vi "Update Command.vi"(6 "Time":dbl, 8 "error in (no error)":errorcluster, 11 "2WayValve in":refnum<class "2WayValveV.lvclass">) -> (0 "error out":errorcluster, 3 "2WayValve out":refnum<class "2WayValveV.lvclass">)   [LabVIEW 2020, in "VolatusGUIElements.lvlib" / "2WayValveV.lvclass"]
uses:
  2WayValveV.lvclass
  2WayValveV.lvclass/2WayValveV.ctl
  lv-vecto/Vecto/Channel DBL/Channel DBL.lvclass/Channel DBL.ctl
  lv-vecto/Vecto/Group DBL/Value by Index.vi
  lv-vecto/Vecto/Channel DBL/Channel DBL.lvclass
  lv-vecto/Vecto/Vecto.lvlib
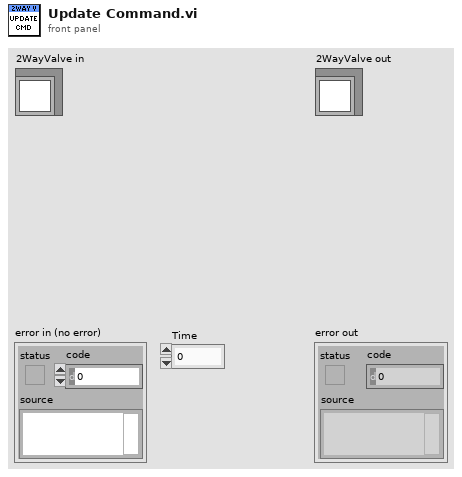
[diagram p1: front panel]
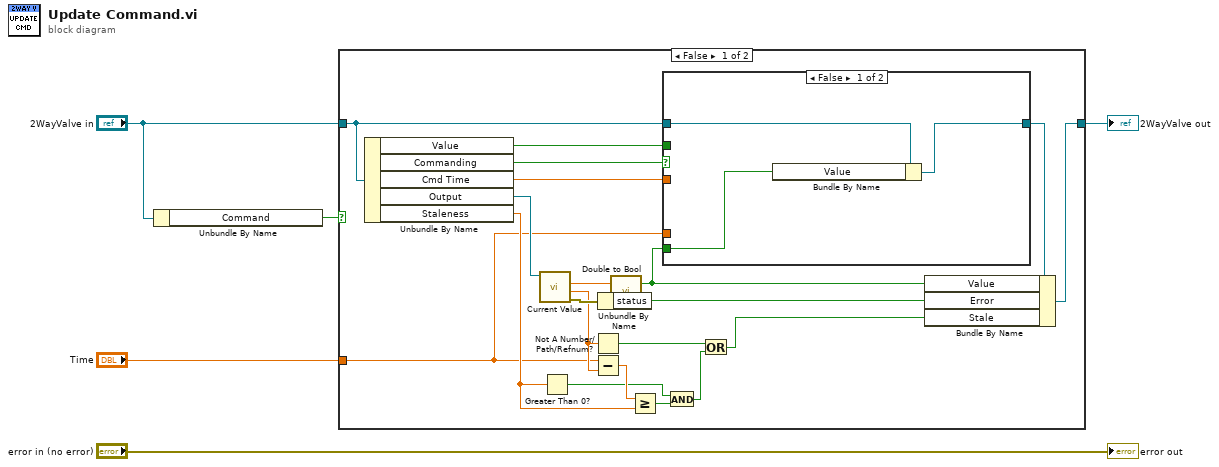
[diagram p0: block diagram]
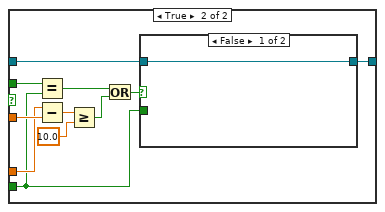
[diagram p2: hidden frame]
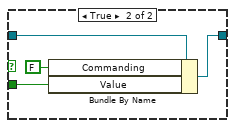
[diagram p3: hidden frame]
diagram:
  n1 = Unbundle By Name("2WayValve in") -> ("Command"=w4:bool)
  n2 = case shown="False" w4 {
    tunnel: [w20 w45] -> w3
    tunnel: "2WayValve in" -> [w8 w45]
    tunnel: "Time" -> [w9 _]
    frame False {
      n3 = Unbundle By Name(w8) -> ("Value"=w10:bool, "Commanding"=w12:bool, "Cmd Time"=w11:dbl, "Output"=w24:refnum<class "Channel DBL.lvclass">, "Staleness"=w19:dbl)
      n4 = call "Current Value.vi"("Channel in"=w24) -> ("error out"=w25:errorcluster, "Timestamp"=w16:dbl, "Scaled"=w23:dbl)  [unwired: 6 in, 2 out]
      n5 = Greater Than 0?(x=w19) -> (x > 0?=w17:bool)
      n6 = Not A Number/Path/Refnum?(number/path/refnum=w16) -> (NaN/Path/Refnum?=w15:bool)
      n7 = Subtract(x=w9, y=w16) -> (x-y=w22:dbl)
      n8 = Unbundle By Name(w25) -> ("status"=w21:bool)
      n9 = call "Double to Bool.vi"("Double"=w23) -> ("Bool"=w7:bool)  [unwired: 2 in]
      n10 = Greater Or Equal?(x=w22, y=w19) -> (x >= y?=w18:bool)
      n11 = case shown="False" w12 {
        tunnel: w11 -> [_ w39]
        tunnel: w10 -> [_ w37]
        tunnel: w9 -> [_ w38]
        tunnel: w8 -> [w28 w32]
        tunnel: w7 -> [w26 w29]
        tunnel: [w27 w31] -> w6
        frame False {
          n12 = Bundle By Name(cluster=w28, "Value"=w26) -> (w27:refnum<class "2WayValveV.lvclass">)
        }
        frame True {
          n13 = Equal?(x=w37, y=w29) -> (x = y?=w36:bool)
          n14 = Subtract(x=w38, y=w39) -> (x-y=w35:dbl)
          n15 = Greater Or Equal?(x=w35, y=10.0) -> (x >= y?=w33:bool)
          n16 = Or(x=w36, y=w33) -> (x .or. y?=w30:bool)
          n17 = case shown="False" w30 {
            tunnel: w32 -> [w40 w44]
            tunnel: [w40 w43] -> w31
            tunnel: w29 -> [_ w41]
            frame False {
            }
            frame True {
              n18 = Bundle By Name(cluster=w44, "Commanding"=FALSE, "Value"=w41) -> (w43:refnum<class "2WayValveV.lvclass">)
            }
          }
        }
      }
      n19 = And(x=w17, y=w18) -> (x .and. y?=w14:bool)
      n20 = Or(x=w15, y=w14) -> (x .or. y?=w13:bool)
      n21 = Bundle By Name(cluster=w6, "Value"=w7, "Error"=w21, "Stale"=w13) -> (w20:refnum<class "2WayValveV.lvclass">)
    }
    frame True {
      # "Command Unused"
    }
  }
  "2WayValve out" <- w3
  "error out" <- "error in (no error)"
